vi "Relation Table Names.vi"(10 "Relation":T1, 11 "Conditum SQLite.lvlib:SQLite.lvclass":refnum<class "SQLite.lvclass">) -> (1 "Reversed By Column Name":string, 2 "Related To Table Name":string)   [LabVIEW 2020, in "Conditum SQLite.lvlib" / "SQLite.lvclass"]
uses:
  SQLite.lvclass
  SQLite.lvclass/SQLite.ctl
  <vilib>/IlluminatedG/IG Conditum Base/Conditum/Relation Mapping.ctl
  <vilib>/IlluminatedG/IG Conditum Base/Conditum/Conditum.lvlib
  <vilib>/IlluminatedG/IG Conditum Base/Conditum/Columns/Relation/Relation Info.ctl
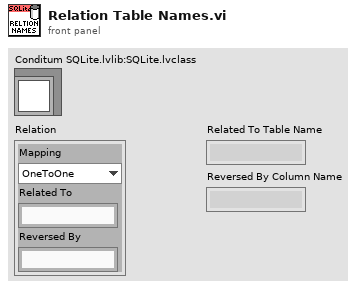
[diagram p1: front panel]
types:
  T1 = typedef "Conditum.lvlib/Relation Info.ctl" = cluster{"Mapping":T2, "Related To":string, "Reversed By":string}
  T2 = typedef "Conditum.lvlib/Relation Mapping.ctl" = enum16{"OneToOne", "OneToMany", "ManyToOne", "ManyToMany"}
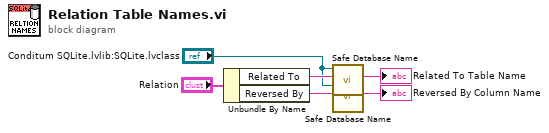
[diagram p0: block diagram]
diagram:
  n1 = Unbundle By Name("Relation") -> ("Related To"=w5:string, "Reversed By"=w4:string)
  n2 = call-dynamic "Safe Database Name.vi"("Conditum Name"=w5, "Database in"="Conditum SQLite.lvlib:SQLite.lvclass") -> ("Database Name"=→"Related To Table Name":string)  [unwired: 9 in]
  n3 = call-dynamic "Safe Database Name.vi"("Conditum Name"=w4, "Database in"="Conditum SQLite.lvlib:SQLite.lvclass") -> ("Database Name"=→"Reversed By Column Name":string)  [unwired: 9 in]
